vi "read_auto_file.vi"(0 "File Name With Extension":string) -> (1 "File Contents":string, 2 "error out":errorcluster)   [LabVIEW 2011]
uses:
  <vilib>/Rock Robotics/WPI/DriverStation/WPI_DriverStationStatusErrorCache.ctl
  <vilib>/Rock Robotics/WPI/DriverStation/DriverStationLCD/WPI_DriverStationLCDLCDLine.ctl
panel:
  out "lowercase file extension":string
  out "file or folder exists?":bool
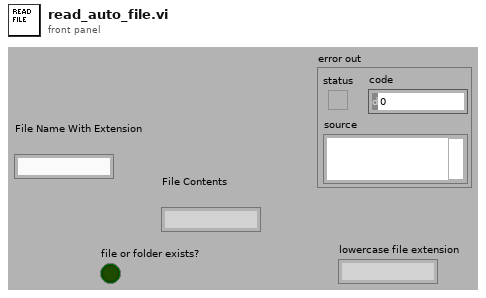
[diagram p1: front panel]
types:
  T1 = typedef "WPI_DriverStationStatusErrorCache.ctl" = enum16{"Get", "Set"}
  T2 = typedef "WPI_DriverStationLCDLCDLine.ctl" = enum16{"Main - Line 1", "User - Line 2", "User - Line 3", "User - Line 4", "User - Line 5", "User - Line 6"}
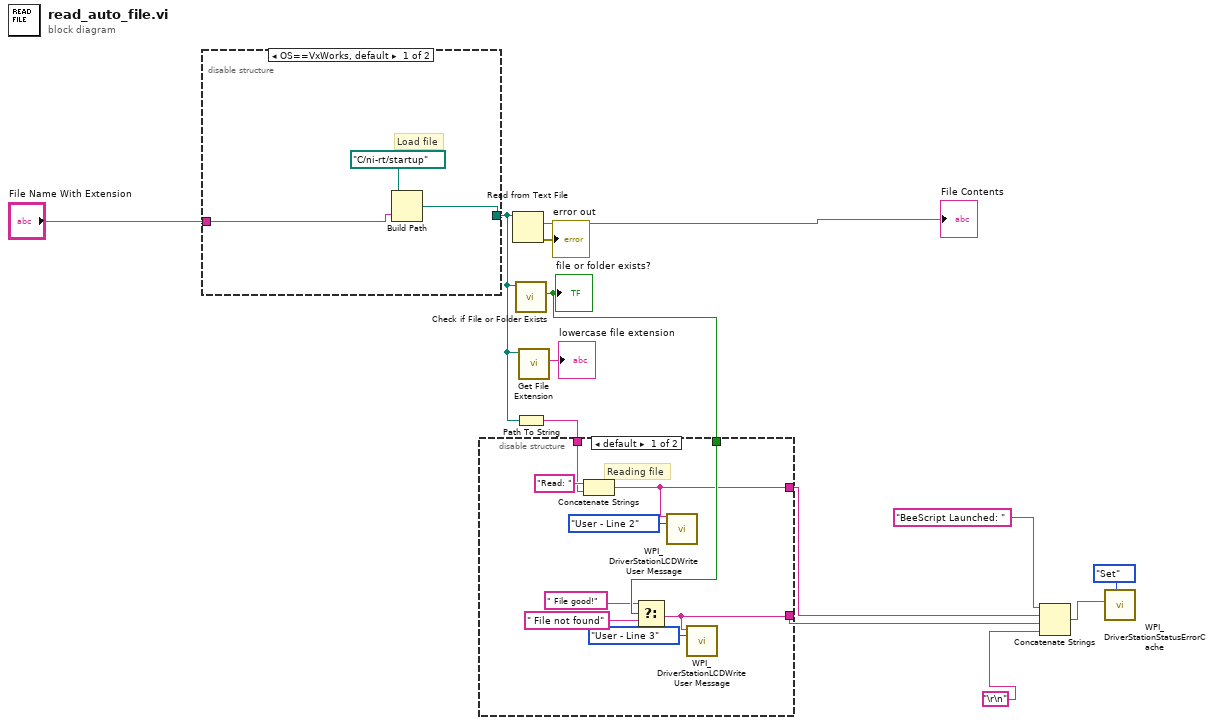
[diagram p0: block diagram]
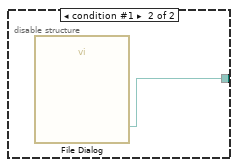
[diagram p3: hidden frame]
diagram:
  n1 = disable-structure shown="OS==VxWorks, default" {
    disable-tunnel: "File Name With Extension" -> [w16 _]
    disable-tunnel: [w14 w17] -> w9
    frame condition #0 (active) {
      # "Load file"
      n2 = Build Path(base path=path "C:/ni-rt/startup", name or relative path=w16) -> (appended path=w14:path)
    }
    frame condition #1 {
      n3 = call "File Dialog"() -> ("selected path"=w17:path)  [unwired: 7 in, 8 out]
    }
  }
  n4 = Read from Text File(file (use dialog)=w9) -> (text=→"File Contents":string, error out=→"error out":errorcluster)  [unwired: 1 in, 4 out]
  n5 = call <vilib>:"Check if File or Folder Exists.vi"("path"=w9) -> ("file or folder exists?"=w10:bool)  [unwired: 1 in, 9 out]
  "file or folder exists?" <- w10
  n6 = Path To String(path=w9) -> (string=w8:string)
  n7 = disable-structure shown="default" {
    disable-tunnel: w10 -> [w24 _]
    disable-tunnel: w8 -> [w20 _]
    disable-tunnel: [w19 _] -> w2
    disable-tunnel: [w18 _] -> w1
    frame condition #0 (active) {
      # "Reading file"
      n8 = Concatenate Strings("Read: " ("string"), w20) -> (w18:string)
      n9 = Select(t=" File good!", s=w24, f=" File not found") -> (s? t:f=w19:string)
      n10 = call <vilib>:"WPI_DriverStationLCDWrite User Message.vi"("line text"=w18, "line"=WPI_DriverStationLCDLCDLine."User - Line 2") -> ()  [unwired: 3 in, 11 out]
      n11 = call <vilib>:"WPI_DriverStationLCDWrite User Message.vi"("line text"=w19, "line"=WPI_DriverStationLCDLCDLine."User - Line 3") -> ()  [unwired: 3 in, 11 out]
    }
    frame condition #1 {
    }
  }
  n12 = call <vilib>:"Get File Extension.vi"("file"=w9) -> ("lowercase file extension"=→"lowercase file extension":string)  [unwired: 1 in, 9 out]
  n13 = Concatenate Strings("BeeScript Launched: " ("string"), w1, w2, "\r\n") -> (w6:string)
  n14 = call <vilib>:"WPI_DriverStationStatusErrorCache.vi"("StatusErrorCacheOp"=WPI_DriverStationStatusErrorCache."Set", "Error String"=w6) -> ()  [unwired: 10 out]
